vi "Stop Core.vi"(10 "final error code":i32, 11 "Chat Window in":refnum<class "Chat Window.lvclass">) -> (3 "Chat Window out":refnum<class "Chat Window.lvclass">)   [LabVIEW 2020, in "Chat Window.lvlib" / "Chat Window.lvclass"]
doc: "(<B>Filename</B>: Actor Framework.lvlib:Actor.lvclass:Stop Core.vi)\n\nDefines what the actor does before it stops. Use the <B>final error code</B> input to determine whether the actor shut down in response to an error.\n\nBy default, this method does nothing. A descendant class may override it to define behavior, such as shutting down any processes the actor initiated in its override of the Actor Core method."
uses:
  Chat Window.lvclass
  Chat Window.lvclass/Chat Window.ctl
  <vilib>/ActorFramework/Actor/Actor.lvclass
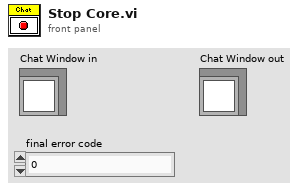
[diagram p1: front panel]
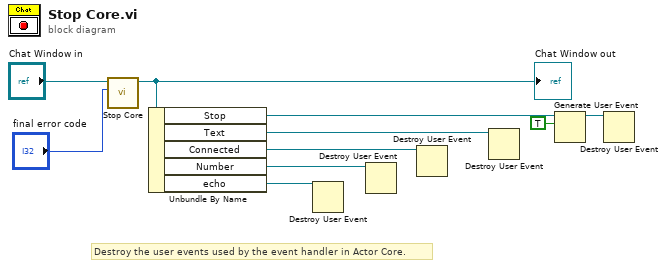
[diagram p0: block diagram]
diagram:
  # "Destroy the user events used by the event handler in Actor Core."
  n1 = call-parent "Stop Core.vi"("final error code"="final error code", "Actor in"="Chat Window in") -> ("Actor out"=w8:refnum<class "Chat Window.lvclass">)  [unwired: 9 in]
  "Chat Window out" <- w8
  n2 = Unbundle By Name(w8) -> ("Stop"=w7:refnum<user-event>, "Text"=w5:refnum<user-event>, "Connected"=w3:refnum<user-event>, "Number"=w2:refnum<user-event>, "echo"=w1:refnum<user-event>)
  n3 = Destroy User Event(user event=w1) -> ()  [unwired: 1 in, 1 out]
  n4 = Destroy User Event(user event=w2) -> ()  [unwired: 1 in, 1 out]
  n5 = Destroy User Event(user event=w3) -> ()  [unwired: 1 in, 1 out]
  n6 = Destroy User Event(user event=w5) -> ()  [unwired: 1 in, 1 out]
  n7 = Generate User Event(user event=w7, event data cluster=TRUE ("event data")) -> (user event out=w4:refnum<user-event>)  [unwired: 2 in, 1 out]
  n8 = Destroy User Event(user event=w4) -> ()  [unwired: 1 in, 1 out]
